vi "filter.vi"(0 "x in":dbl[](array[numeric]), 7 "y in":dbl[](array[numeric]), 11 "z in":dbl[](array[numeric]), 12 "Threshold min":dbl, 13 "Threshold max":dbl) -> (4 "x out":dbl[](array[numeric]), 8 "y out":dbl[](array[numeric]), 15 "z out":dbl[](array[numeric]))   [LabVIEW 2023]
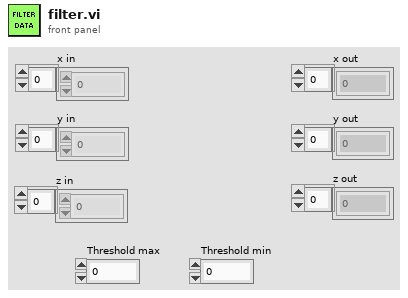
[diagram p1: front panel]
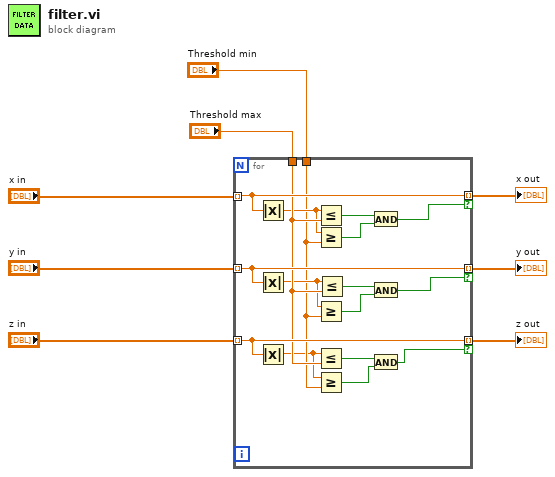
[diagram p0: block diagram]
diagram:
  n1 = for {
    tunnel: "x in" -> [w25] mode=indexing
    tunnel: "y in" -> [w24] mode=indexing
    tunnel: "z in" -> [w23] mode=indexing
    tunnel: "Threshold max" -> [w22]
    tunnel: [w25] -> w6 mode=indexing if=w18
    tunnel: [w24] -> w7 mode=indexing if=w13
    tunnel: [w23] -> w8 mode=indexing if=w9
    tunnel: "Threshold min" -> [w15]
    n2 = Absolute Value(x=w25) -> (abs(x)=w19:dbl)
    n3 = Absolute Value(x=w24) -> (abs(x)=w16:dbl)
    n4 = Absolute Value(x=w23) -> (abs(x)=w14:dbl)
    n5 = Less Or Equal?(x=w19, y=w22) -> (x <= y?=w20:bool)
    n6 = Greater Or Equal?(x=w19, y=w15) -> (x >= y?=w17:bool)
    n7 = Greater Or Equal?(x=w16, y=w15) -> (x >= y?=w12:bool)
    n8 = Less Or Equal?(x=w14, y=w22) -> (x <= y?=w11:bool)
    n9 = Greater Or Equal?(x=w14, y=w15) -> (x >= y?=w10:bool)
    n10 = Less Or Equal?(x=w16, y=w22) -> (x <= y?=w21:bool)
    n11 = And(x=w20, y=w17) -> (x .and. y?=w18:bool)
    n12 = And(x=w21, y=w12) -> (x .and. y?=w13:bool)
    n13 = And(x=w11, y=w10) -> (x .and. y?=w9:bool)
  }
  "z out" <- w8
  "y out" <- w7
  "x out" <- w6
